vi "Is Using GH2.vi"(8 "error in (no error)":errorcluster, 11 "Gantry in":refnum<class "Gantry.lvclass">) -> (0 "error out":errorcluster, 2 "Using GH2":bool, 3 "Gantry out":refnum<class "Gantry.lvclass">)   [LabVIEW 2026, in "Gantry.lvclass"]
uses:
  Gantry.lvclass
  Gantry.lvclass/Gantry.ctl
  FlexWorktable/FlexWorktable.lvclass
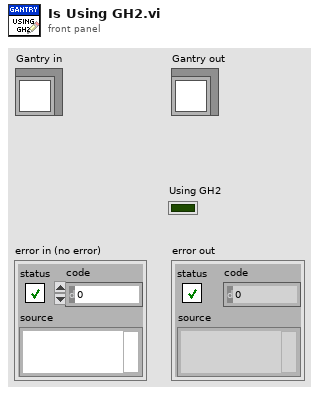
[diagram p1: front panel]
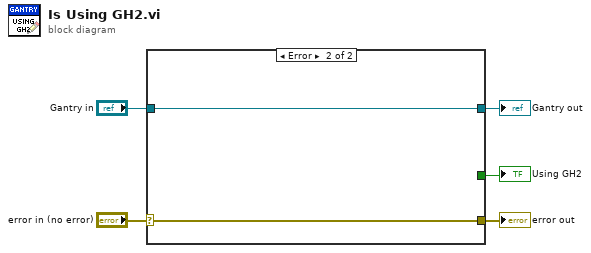
[diagram p0: block diagram]
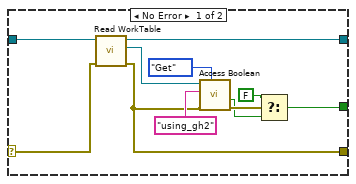
[diagram p2: hidden frame]
diagram:
  n1 = case shown="Error" "error in (no error)" {
    selector: "error in (no error)" -> [w14 w18]
    tunnel: [w6 w18] -> w4
    tunnel: [w15 w17] -> w2
    tunnel: "Gantry in" -> [w16 w17]
    tunnel: [w7 _] -> w1
    frame No Error {
      n2 = call-dynamic "Read WorkTable.vi"("error in"=w14, "Gantry Class in"=w16) -> ("error out"=w6:errorcluster, "Worktable"=w13:refnum<class "FlexWorktable.lvclass">, "Gantry Class out"=w15:refnum<class "Gantry.lvclass">)  [unwired: 7 in]
      n3 = call-dynamic "Access Boolean.vi"("Get/Set"=enum16{"Get", "Set"}."Get", "error in (no error)"=w6, "Key"="using_gh2", "FlexWorktable in"=w13) -> ("error out"=w10:errorcluster, "Value out"=w8:bool)  [unwired: 5 in, 1 out]
      n4 = Select(t=FALSE, s=w10, f=w8) -> (s? t:f=w7:bool)
    }
    frame Error {
    }
  }
  "error out" <- w4
  "Gantry out" <- w2
  "Using GH2" <- w1
